vi "File Existence.vi"(1 "Path":path) -> (0 "exists":bool, 2 "is directory":bool)   [LabVIEW 2018]
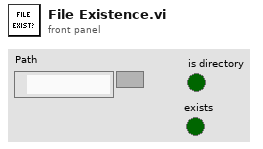
[diagram p1: front panel]
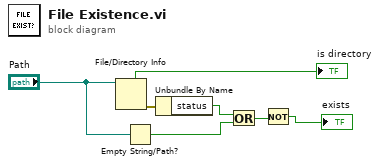
[diagram p0: block diagram]
diagram:
  n1 = File/Directory Info(path="Path") -> (directory=→"is directory":bool, error out=w7:errorcluster)  [unwired: 1 in, 5 out]
  n2 = Empty String/Path?(string/path="Path") -> (empty?=w3:bool)
  n3 = Unbundle By Name(w7) -> ("status"=w4:bool)
  n4 = Or(x=w4, y=w3) -> (x .or. y?=w2:bool)
  n5 = Not(x=w2) -> (.not. x?=→"exists":bool)
